vi "SP Format Value to Fundamental (array).vi"(4 "Sxx Display Format":T1, 5 "Display Values":dbl[](array[numeric])) -> (1 "Stored Values":dbl[](array[numeric]))   [LabVIEW 2011]
uses:
  TypeDefs/SP Format.ctl
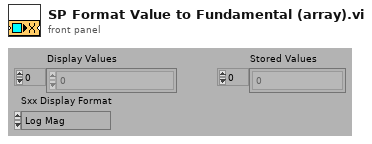
[diagram p1: front panel]
types:
  T1 = typedef "SP Format.ctl" = enum16{"Log Mag", "Lin Mag", "SWR", "Phase", "Expanded Phase", "Delay", "Insertion Loss", "Isolation", "Return Loss"}
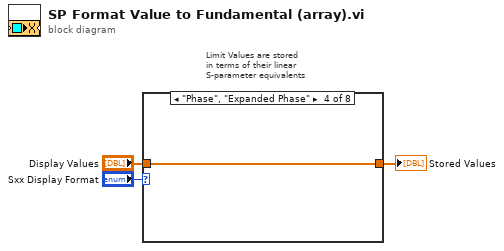
[diagram p0: block diagram]
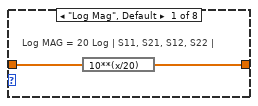
[diagram p2: hidden frame]
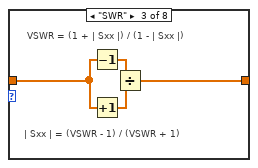
[diagram p4: hidden frame]
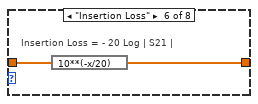
[diagram p6: hidden frame]
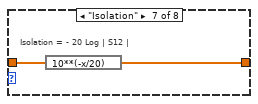
[diagram p7: hidden frame]
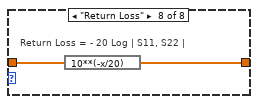
[diagram p8: hidden frame]
diagram:
  # "Limit Values are stored\nin terms of their linear\nS-parameter equivalents"
  n1 = case shown="\"Phase\", \"Expanded Phase\"" "Sxx Display Format" {
    tunnel: [w5 w6 w9 w11 w12 w13 w15 w17] -> w1
    tunnel: "Display Values" -> [w4 w6 w8 w11 w12 w14 w16 w18]
    frame "Log Mag", Default {
      # "Log MAG = 20 Log | S11, S21, S12, S22 |"
      n2 = expression code="10**(x/20)"(w4) -> (w5:dbl[])
    }
    frame "Lin Mag" {
    }
    frame "SWR" {
      # "| Sxx | = (VSWR - 1) / (VSWR + 1)"
      # "VSWR = (1 + | Sxx |) / (1 - | Sxx |)"
      n3 = Decrement(x=w8) -> (x-1=w10:dbl[])
      n4 = Increment(x=w8) -> (x+1=w7:dbl[])
      n5 = Divide(x=w10, y=w7) -> (x/y=w9:dbl[])
    }
    frame "Phase", "Expanded Phase" {
    }
    frame "Delay" {
      # "Group Delay is a derived quantity - we save \nthe number as is..."
    }
    frame "Insertion Loss" {
      # "Insertion Loss = - 20 Log | S21 |"
      n6 = expression code="10**(-x/20)"(w14) -> (w13:dbl[])
    }
    frame "Isolation" {
      # "Isolation = - 20 Log | S12 |"
      n7 = expression code="10**(-x/20)"(w16) -> (w15:dbl[])
    }
    frame "Return Loss" {
      # "Return Loss = - 20 Log | S11, S22 |"
      n8 = expression code="10**(-x/20)"(w18) -> (w17:dbl[])
    }
  }
  "Stored Values" <- w1
